vi "write_error_time.vi"(10 "error_time":timestamp, 11 "Error in":refnum<class "Error.lvclass">) -> (3 "Error out":refnum<class "Error.lvclass">)   [LabVIEW 2023, in "Error Handling Interface.lvlib" / "Error.lvclass"]
uses:
  Error.lvclass
  Error.lvclass/Error.ctl
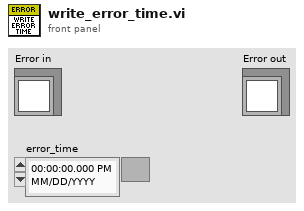
[diagram p1: front panel]
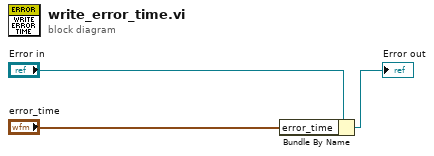
[diagram p0: block diagram]
diagram:
  n1 = Bundle By Name(cluster="Error in", "error_time"="error_time") -> (→"Error out":refnum<class "Error.lvclass">)
